vi "Copy Gplugin datafile.vi"(11 "error in (no error)":errorcluster) -> (15 "error out":errorcluster)   [LabVIEW 2021, in "G Plug-in Migrator.lvlib"]
uses:
  G Plug-in Migrator.lvlib
  Migrator Reusables/Migrator Reusables.lvlib
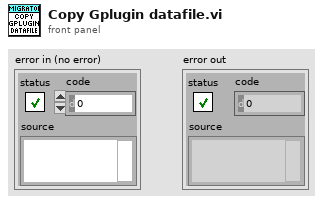
[diagram p1: front panel]
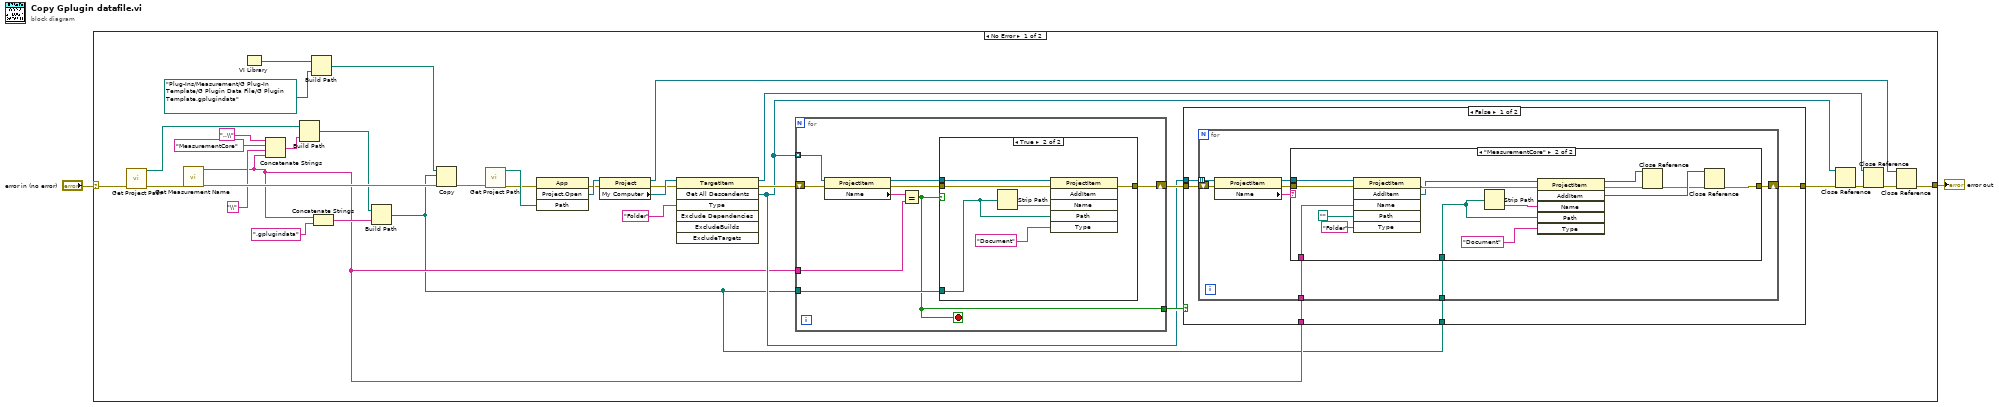
[diagram p0: block diagram]
diagram:
  n1 = case shown="No Error" "error in (no error)" {
    selector: "error in (no error)" -> [w30 w83]
    tunnel: [w9 w83] -> w2
    frame No Error {
      n2 = call "Get Project Path.vi"("error in (no error)"=w30) -> ("Project Path Out"=w28:path, "error out"=w29:errorcluster)  [unwired: 13 in]
      n3 = call "Get Measurement Name.vi"("error in (no error)"=w29) -> ("Name Out"=w5:string, "error out"=w31:errorcluster)  [unwired: 13 in]
      n4 = VI Library() -> (path=w36:path)
      n5 = Concatenate Strings("..\\" ("string"), "MeasurementCore" ("string"), "\\" ("string"), w5) -> (w25:string)
      n6 = Build Path(base path=w28, name or relative path=w25) -> (appended path=w24:path)
      n7 = Build Path(base path=w36, name or relative path=path "Plug-Ins/Measurement/G Plug-In Template/G Plugin Data File/G Plugin Template.gplugindata") -> (appended path=w32:path)
      n8 = Concatenate Strings(w5, ".gplugindata" ("string")) -> (w33:string)
      n9 = Build Path(base path=w24, name or relative path=w33) -> (appended path=w4:path)
      n10 = Copy(8:w31, 10:w4, 11:w32) -> (0:w20:errorcluster)  [unwired: 2 in, 2 out]
      n11 = call "Get Project Path.vi"("error in (no error)"=w20) -> ("Project Path Out"=w22:path, "error out"=w21:errorcluster)  [unwired: 13 in]
      n12 = invoke class="App" method="Project.Open"(error in=w21, "Path"=w22) -> (error out=w16:errorcluster, "Project:Open"=w18:refnum<vi>)  [unwired: 2 in, 2 out]
      n13 = property class="Project"(reference=w18, error in=w16) -> (reference out=w10:refnum<vi>, error out=w15:errorcluster, "My Computer"=w17:refnum<vi>)
      n14 = invoke class="TargetItem" method="Get All Descendents"(reference=w17, error in=w15, "Type"="Folder") -> (reference out=w12:refnum<vi>, error out=w14:errorcluster, "All Descendents"=w6:refnum<vi>[])  [unwired: 4 in, 4 out]
      n15 = for {
        tunnel: w6 -> [w75] mode=indexing
        tunnel: w5 -> [w72]
        tunnel: w4 -> [w69]
        shift-right: [w68] -> w7
        shift-left: w14 -> [w74]
        tunnel: [w67] -> w8
        stop <- w67 stop-if-true
        n16 = property class="ProjectItem"(reference=w75, error in=w74) -> (reference out=w70:refnum<vi>, error out=w71:errorcluster, "Name"=w73:string)
        n17 = Equal?(x=w73, y=w72) -> (x = y?=w67:bool)
        n18 = case shown="True" w67 {
          tunnel: w71 -> [w76 w79]
          tunnel: w70 -> [_ w80]
          tunnel: w69 -> [_ w78]
          tunnel: [w76 w77] -> w68
          frame False {
          }
          frame True {
            n19 = Strip Path(path=w78) -> (name=w81:string)  [unwired: 1 out]
            n20 = invoke class="ProjectItem" method="AddItem"(reference=w80, error in=w79, "Name"=w81, "Path"=w78, "Type"="Document") -> (error out=w77:errorcluster)  [unwired: 1 in, 5 out]
          }
        }
      }
      n21 = case shown="False" w8 {
        tunnel: w7 -> [w40 w66]
        tunnel: w6 -> [w41 _]
        tunnel: w5 -> [w39 _]
        tunnel: w4 -> [w38 _]
        tunnel: [w37 w66] -> w3
        frame False {
          n22 = for {
            tunnel: w41 -> [w48] mode=indexing
            tunnel: w39 -> [w44]
            tunnel: w38 -> [w43]
            shift-right: [w42] -> w37
            shift-left: w40 -> [w49]
            n23 = property class="ProjectItem"(reference=w48, error in=w49) -> (reference out=w45:refnum<vi>, error out=w46:errorcluster, "Name"=w47:string)
            n24 = case shown="\"MeasurementCore\"" w47 {
              tunnel: w46 -> [w50 w64]
              tunnel: w45 -> [_ w65]
              tunnel: w44 -> [_ w63]
              tunnel: w43 -> [_ w57]
              tunnel: [w50 w55] -> w42
              frame Default {
              }
              frame "MeasurementCore" {
                n25 = invoke class="ProjectItem" method="AddItem"(reference=w65, error in=w64, "Name"=w63, "Path"=path "", "Type"="Folder") -> (error out=w58:errorcluster, "AddItem"=w53:refnum<vi>)  [unwired: 1 in, 4 out]
                n26 = Strip Path(path=w57) -> (name=w60:string)  [unwired: 1 out]
                n27 = invoke class="ProjectItem" method="AddItem"(reference=w53, error in=w58, "Name"=w60, "Path"=w57, "Type"="Document") -> (reference out=w51:refnum<vi>, error out=w56:errorcluster, "AddItem"=w54:refnum<vi>)  [unwired: 1 in, 3 out]
                n28 = Close Reference(reference=w51, error in (no error)=w56) -> (error out=w52:errorcluster)
                n29 = Close Reference(reference=w54, error in (no error)=w52) -> (error out=w55:errorcluster)
              }
            }
          }
        }
        frame True {
        }
      }
      n30 = Close Reference(reference=w6, error in (no error)=w3) -> (error out=w13:errorcluster)
      n31 = Close Reference(reference=w12, error in (no error)=w13) -> (error out=w11:errorcluster)
      n32 = Close Reference(reference=w10, error in (no error)=w11) -> (error out=w9:errorcluster)
    }
    frame Error {
    }
  }
  "error out" <- w2
